vi "R-einfach invers LQR.vi"(8 "Winkelgeschwindigkeit":dbl, 9 "Winkel":dbl, 10 "Geschwindigkeit":dbl, 11 "Position":dbl) -> (2 "Stellgröße":dbl)   [LabVIEW 2014]
panel:
  in  "k 4":dbl
  in  "k 3":dbl
  in  "k 2":dbl
  in  "k 1":dbl
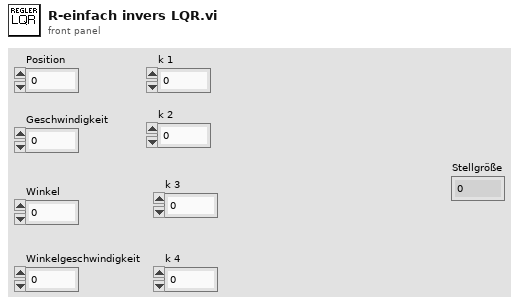
[diagram p1: front panel]
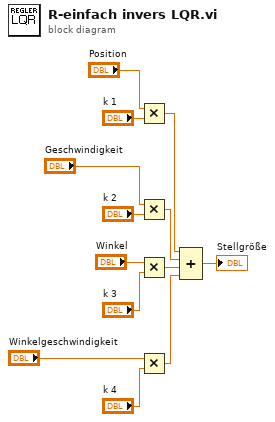
[diagram p0: block diagram]
diagram:
  n1 = Multiply(x="Position", y="k 1") -> (x*y=w1:dbl)
  n2 = Multiply(x="Geschwindigkeit", y="k 2") -> (x*y=w2:dbl)
  n3 = Multiply(x="Winkel", y="k 3") -> (x*y=w3:dbl)
  n4 = Multiply(x="Winkelgeschwindigkeit", y="k 4") -> (x*y=w4:dbl)
  n5 = Compound Arithmetic op=ADD(w1, w2, w3, w4) -> (→"Stellgröße":dbl)
